vi "Host.vi"() -> ()   [LabVIEW 2018]
uses:
  <instrlib>/niDMM/nidmm.llb/niDMM Resolution in Digits.ctl
  <instrlib>/niDMM/nidmm.llb/niDMM Function.ctl
  <instrlib>/niDCPower/nidcpower.llb/niDCPower Measurement Type.ctl
  <instrlib>/niScope/Configure/Trigger/niScope Configure Trigger Edge.vi
  <instrlib>/niScope/Acquire/Fetch/niScope Multi Fetch Cluster.vi
  <instrlib>/niScope/Acquire/Fetch/niScope Fetch.vi
  <instrlib>/niDMM/nidmm.llb/niDMM Configure Measurement Digits.vi
panel:
  in  "Tab Control":enum32{"Панель управления", "Панель отладки"}(tab)
  out "Образец №":string="0"
  in  "SEL":path=path "D:/NI LabVIEW/21.057 MAX3738ETG+/SEL and SEU"
  out "VCC_char":dbl(graph)=6.67426339573744e-05
  in  "VCC, V":dbl=3.300000000000001 caption="voltage level" format="%_6p"
  out "VCC_cur, A":dbl=6.67426339573744e-05 caption="measurement" format="%_6g"
  in  "VCC_curlim, A":dbl=0.1 caption="current limit" format="%_6p"
  out "VCC_warning":bool
  in  "VCC_selcur, A":dbl=0.07 caption="current limit" format="%_6p"
  out "VCC_counter":u32
  out "SEL":bool
  out "SEU":bool
  in  "POWER":bool
  in  "Device Name":refnum<k15>="PXI1Slot6_3" caption="DMM (BIAS current)"
  in  "POWER (0 KEY(GND), 1 PRBS)":refnum<k15>="PXI1Slot3_3" caption="PRBS"
  in  "PRBS":bool
  in  "RELAY":bool
  in  "NI Scope (SHUTDOWN)":refnum<k15>="PXI1Slot5_2" caption="Scope"
  in  "POWER (0 VСС, 1 +5)":refnum<k15>="PXI1Slot2_2" caption="VСС_+5"
  out "DIOD, мA":dbl=0.00012235000212967861 caption="measurement" format="%_6g"
  out "SEU Waveform":T1(graph) caption="SHUTDOWN Waveform"
  in  "Trigger Level":dbl=2.9 format="%.2f"
  in  "Диапазон, A":dbl=0.1 caption="voltage level" format="%_6p"
  out "BC_MON_char":dbl(graph)=6.67426339573744e-05
  out "SEU_Counter":u32 caption="SEU counter"
  out "SEU_warning":bool caption="Find SEL"
  out "+5_char":dbl(graph)=4.2515020717360033e-07
  in  "+5, V":dbl=5.0 caption="voltage level" format="%_6p"
  out "+5_cur, A":dbl=4.2515020717360033e-07 caption="measurement" format="%_6g"
  in  "+5_curlim, A":dbl=0.1 caption="current limit" format="%_6p"
  out "PRBS_char":dbl(graph)=8.696388929340759e-07
  in  "PRBS, V":dbl=12.0 caption="voltage level" format="%_6p"
  out "PRBS_cur, A":dbl=8.696388929340759e-07 caption="measurement" format="%_6g"
  in  "PRBS_curlim, A":dbl=0.1 caption="current limit" format="%_6p"
  in  "SIM_SEL":bool
  in  "STOP":bool
  in  "Парирование SEU":bool=TRUE
  in  "Антизалип":bool=TRUE
  in  "POWER (0 DIOD, 1 TX_DISABLE)":refnum<k15>="PXI1Slot4_3" caption="PRBS"
  out "SHUTDOWN Waveform":T1(graph) caption="PC_MON Waveform"
  in  "DIOD_curlim, A":dbl=0.025 caption="current limit" format="%_6p"
  out "DIOD_cur, A":dbl=6.67426339573744e-05 caption="measurement" format="%_6g"
  in  "DIOD, V":dbl=3.300000000000001 caption="voltage level" format="%_6p"
  out "DIOD_char":dbl(graph)=6.67426339573744e-05
  in  "TX_DISABLE":bool
  in  "DIOD":bool
  in  "IN1(GND)":bool
  in  "IN1(GND)_curlim, A":dbl=0.01 caption="current limit" format="%_6p"
  out "IN1(GND)_cur, A":dbl=8.696388929340759e-07 caption="measurement" format="%_6g"
  in  "IN1(GND), V":dbl=3.3 caption="voltage level" format="%_6p"
  in  "TX_DISABLE_curlim, A":dbl=0.01 caption="current limit" format="%_6p"
  in  "TX_DISABLE, V":dbl=3.3 caption="voltage level" format="%_6p"
  out "TX_DISABLE_cur, A":dbl=8.696388929340759e-07 caption="measurement" format="%_6g"
  in  "SEU":path=path "D:/NI LabVIEW/21.057 MAX3738ETG+/SEL and SEU"
  out "Power OFF":bool
  in  "VCC ON":bool
  in  "Считать Ключ":bool
  in  "Считать SIM_SEL":bool
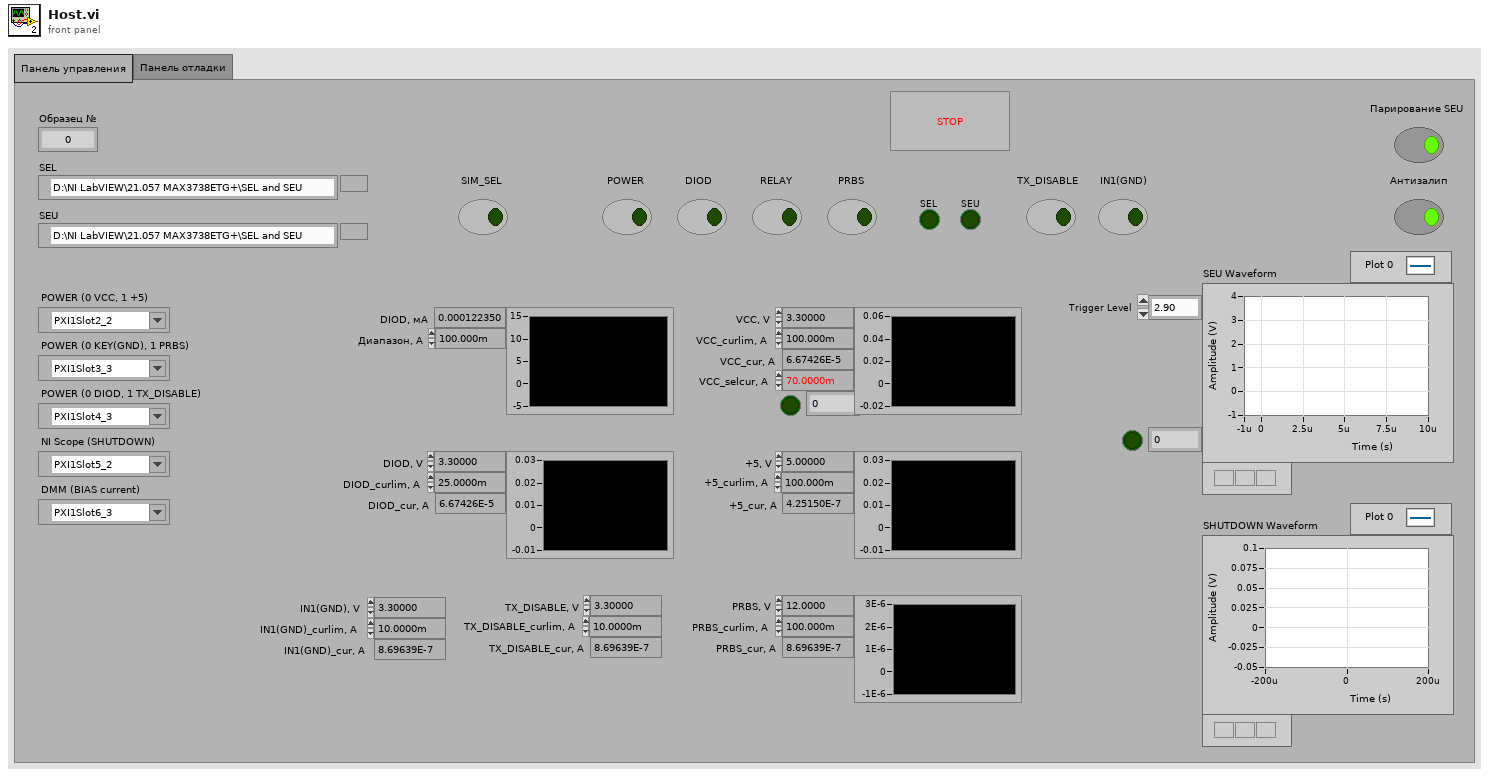
[diagram p1: front panel]
types:
  T1 = cluster{"relativeInitialX":dbl, "xIncrement":dbl, "wfm":dbl[]}[]
  T2 = enum16{"open", "replace", "create", "open or create", "replace or create", "replace or create with confirmation"}
  T3 = typedef "niDCPower Measurement Type.ctl" = i32
  T4 = typedef "niDMM Function.ctl" = enum16{"DC Volts", "AC Volts", "DC Current", "AC Current", "2-wire Resistance", "4-wire Resistance", "Diode", "Frequency", "Period", "AC Volts DC Coupled", "Capacitance", "Inductance", "Temperature"}
  T5 = typedef "niDMM Resolution in Digits.ctl" = dbl
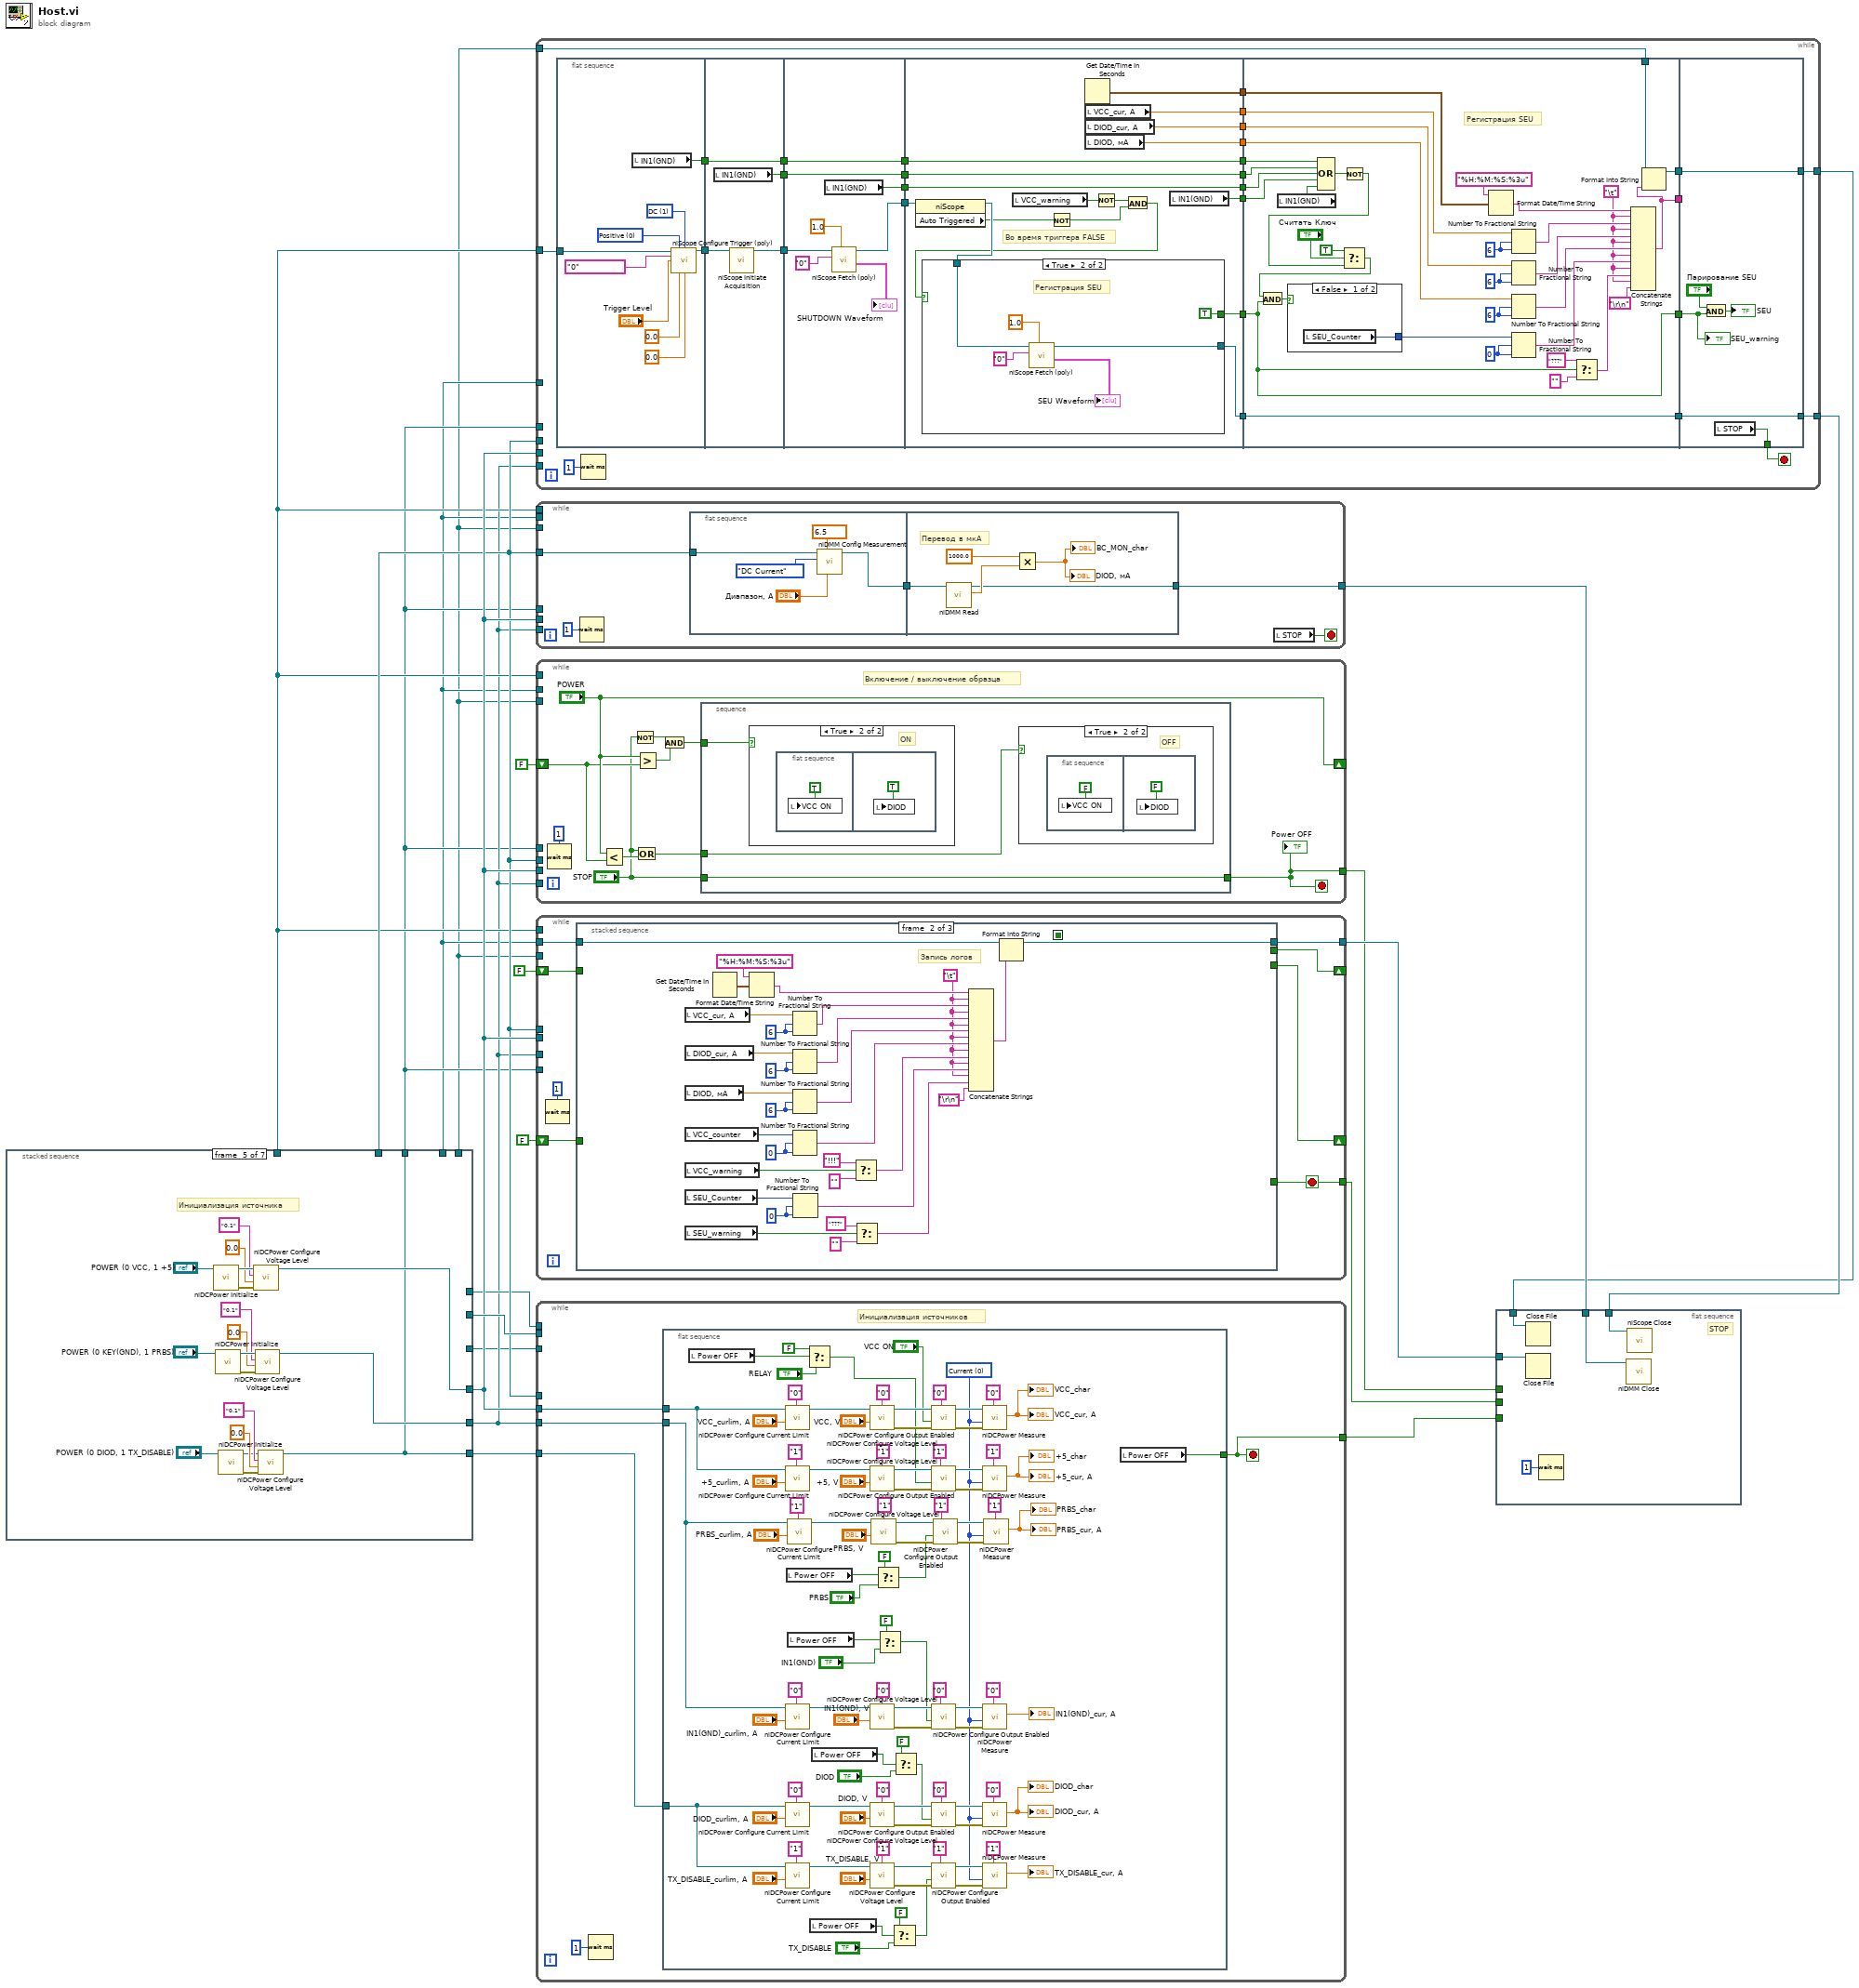
[diagram p0: block diagram]
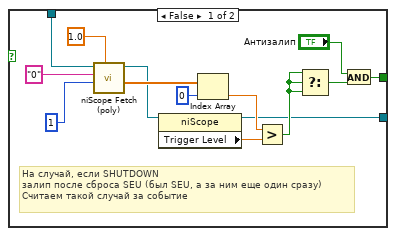
[diagram p2: hidden frame]
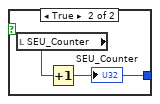
[diagram p3: hidden frame]
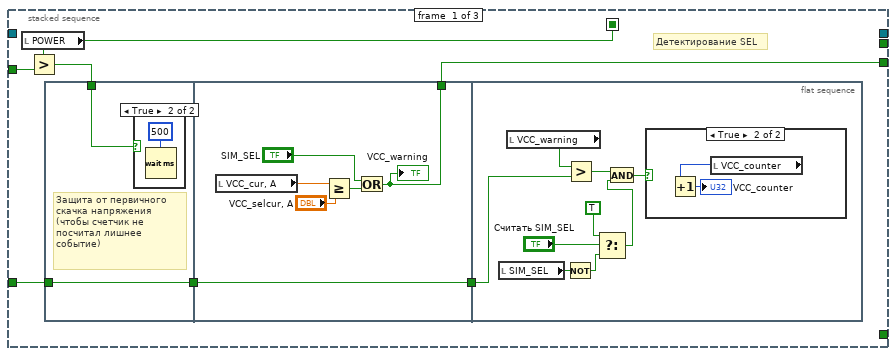
[diagram p4: hidden frame]
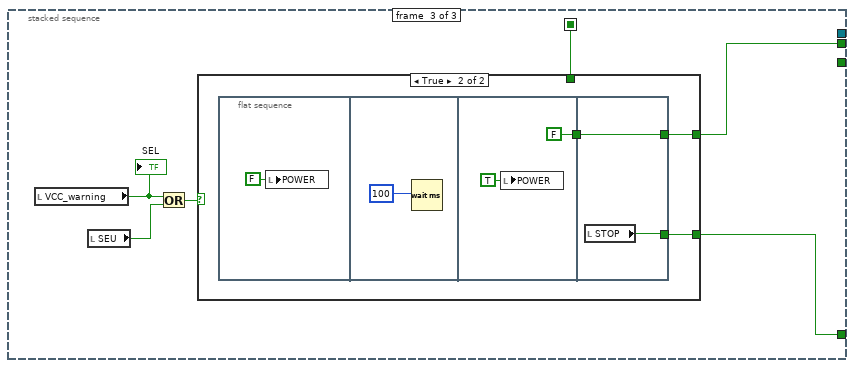
[diagram p7: hidden frame]
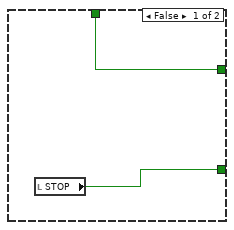
[diagram p8: hidden frame]
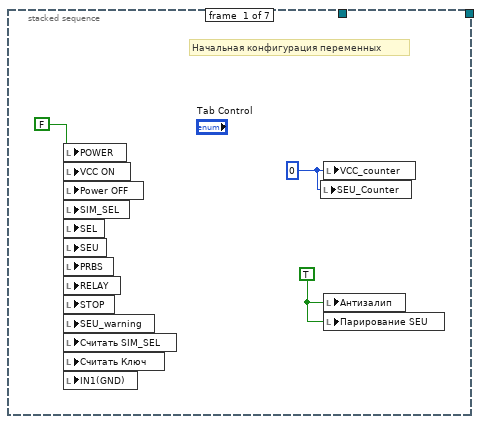
[diagram p11: hidden frame]
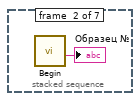
[diagram p12: hidden frame]
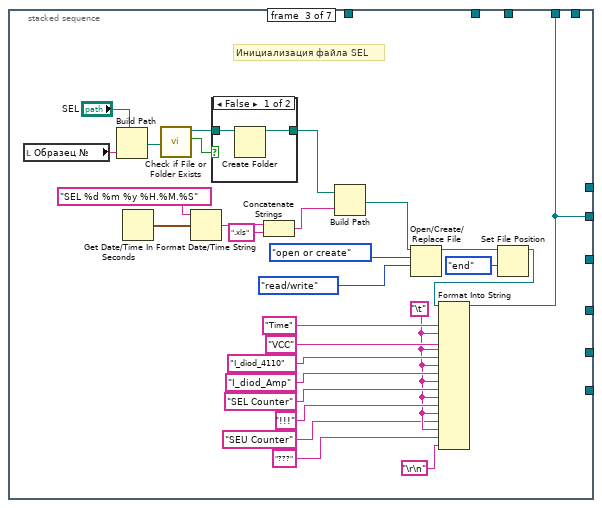
[diagram p13: hidden frame]
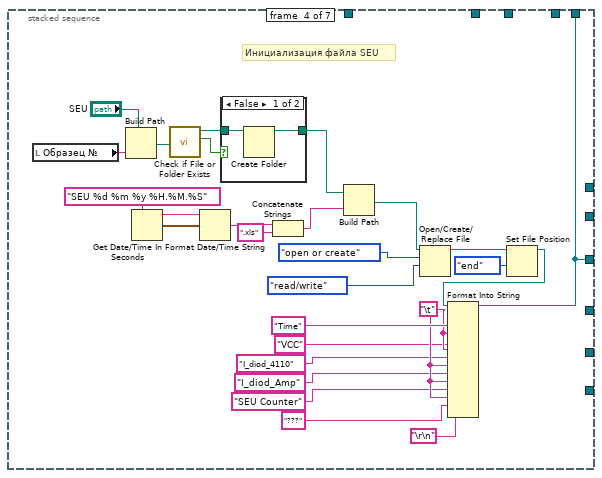
[diagram p15: hidden frame]
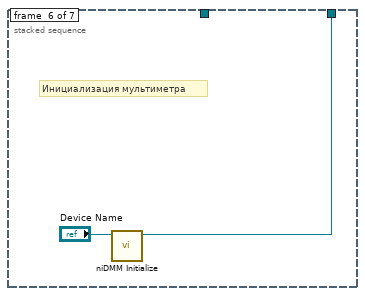
[diagram p17: hidden frame]
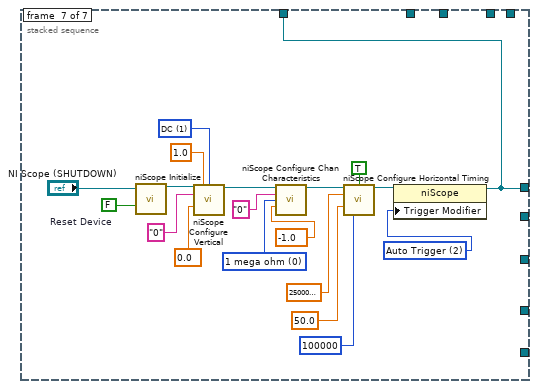
[diagram p18: hidden frame]
diagram:
  n1 = stacked-sequence {
    tunnel: [_ _ _ _ w99 _ _] -> w12
    tunnel: [_ _ w34 _ _ _ _] -> w4
    tunnel: [_ _ w34 _ _ _ _] -> w18
    tunnel: [_ _ _ _ _ w104 _] -> w11
    tunnel: [_ _ _ _ w92 _ _] -> w7
    tunnel: [_ _ _ _ _ _ w106] -> w10
    tunnel: [_ _ _ _ _ _ w106] -> w9
    tunnel: [_ _ _ _ w86 _ _] -> w6
    tunnel: [_ _ _ _ w86 _ _] -> w5
    tunnel: [_ _ _ w57 _ _ _] -> w3
    tunnel: [_ _ _ w57 _ _ _] -> w2
    frame #0 {
      w23 = TRUE ("Питание")
      w24 = u32 0 ("VCC_counter")
      w22 = FALSE ("Питание")
      # "Начальная конфигурация переменных"
      n2 = local write "POWER"(w22) -> ()
      n3 = local write "VCC ON"(w22) -> ()
      n4 = local write "Power OFF"(w22) -> ()
      n5 = local write "SIM_SEL"(w22) -> ()
      n6 = local write "SEL"(w22) -> ()
      n7 = local write "SEU"(w22) -> ()
      n8 = local write "PRBS"(w22) -> ()
      n9 = local write "RELAY"(w22) -> ()
      n10 = local write "STOP"(w22) -> ()
      n11 = local write "SEU_warning"(w22) -> ()
      n12 = local write "Считать SIM_SEL"(w22) -> ()
      n13 = local write "Считать Ключ"(w22) -> ()
      n14 = local write "IN1(GND)"(w22) -> ()
      n15 = local write "SEU_Counter"(w24) -> ()
      n16 = local write "VCC_counter"(w24) -> ()
      n17 = local write "Антизалип"(w23) -> ()
      n18 = local write "Парирование SEU"(w23) -> ()
    }
    frame #1 {
      n19 = call "Begin.vi"() -> ("Образец № 2"=→"Образец №":string)  [unwired: 9 in]
    }
    frame #2 {
      w29 = "\t"
      # "Инициализация файла SEL"
      n20 = local read "Образец №"() -> (w36:string)
      n21 = Build Path(base path="SEL", name or relative path=w36) -> (appended path=w53:path)
      n22 = Get Date/Time In Seconds() -> (seconds since 1Jan1904=w49:timestamp)
      n23 = call <vilib>:"Check if File or Folder Exists.vi"("path"=w53) -> ("file or folder exists?"=w52:bool, "dup path"=w51:path)  [unwired: 8 in, 1 out]
      n24 = Format Date/Time String(time format string (%c)="SEL %d %m %y %H.%M.%S", seconds (now)=w49) -> (date/time string=w48:string)  [unwired: 1 in]
      n25 = case shown="False" w52 {
        tunnel: w51 -> [w55 w56]
        tunnel: [w54 w56] -> w50
        frame False {
          n26 = Create Folder(path (use dialog)=w55) -> (created path=w54:path)  [unwired: 2 in, 2 out]
        }
        frame True {
        }
      }
      n27 = Concatenate Strings(w48, ".xls" ("string")) -> (w45:string)
      n28 = Build Path(base path=w50, name or relative path=w45) -> (appended path=w42:path)
      n29 = Open/Create/Replace File(file path (use dialog)=w42, operation (0:open)=T2."open or create", access (0:read/write)=enum16{"read/write", "read-only", "write-only"}."read/write") -> (refnum out=w39:refnum<file>)  [unwired: 3 in, 2 out]
      n30 = Set File Position(refnum=w39, from (0:start)=enum16{"start", "end", "current"}."end") -> (refnum out=w35:refnum<file>)  [unwired: 2 in, 1 out]
      n31 = Format Into String(initial string=w35, "Time" ("string"), w29, "VCC" ("string"), w29, "I_diod_4110" ("string"), w29, "I_diod_Amp" ("input 7"), w29, "SEL Counter" ("string"), w29, "!!!" ("string"), w29, "SEU Counter" ("string"), w29, "???" ("string"), "\r\n") -> (resulting string=w34:refnum<file>)  [unwired: 2 in, 1 out]
    }
    frame #3 {
      w69 = "\t"
      # "Инициализация файла SEU"
      n32 = local read "Образец №"() -> (w72:string)
      n33 = Build Path(base path="SEU", name or relative path=w72) -> (appended path=w82:path)
      n34 = Get Date/Time In Seconds() -> (seconds since 1Jan1904=w78:timestamp)
      n35 = call <vilib>:"Check if File or Folder Exists.vi"("path"=w82) -> ("file or folder exists?"=w81:bool, "dup path"=w80:path)  [unwired: 8 in, 1 out]
      n36 = Format Date/Time String(time format string (%c)="SEU %d %m %y %H.%M.%S", seconds (now)=w78) -> (date/time string=w77:string)  [unwired: 1 in]
      n37 = case shown="False" w81 {
        tunnel: w80 -> [w84 w85]
        tunnel: [w83 w85] -> w79
        frame False {
          n38 = Create Folder(path (use dialog)=w84) -> (created path=w83:path)  [unwired: 2 in, 2 out]
        }
        frame True {
        }
      }
      n39 = Concatenate Strings(w77, ".xls" ("string")) -> (w76:string)
      n40 = Build Path(base path=w79, name or relative path=w76) -> (appended path=w75:path)
      n41 = Open/Create/Replace File(file path (use dialog)=w75, operation (0:open)=T2."open or create", access (0:read/write)=enum16{"read/write", "read-only", "write-only"}."read/write") -> (refnum out=w74:refnum<file>)  [unwired: 3 in, 2 out]
      n42 = Set File Position(refnum=w74, from (0:start)=enum16{"start", "end", "current"}."end") -> (refnum out=w58:refnum<file>)  [unwired: 2 in, 1 out]
      n43 = Format Into String(initial string=w58, "Time" ("string"), w69, "VCC" ("string"), w69, "I_diod_4110" ("string"), w69, "I_diod_Amp" ("input 7"), w69, "SEU Counter" ("string"), w69, "???" ("string"), "\r\n") -> (resulting string=w57:refnum<file>)  [unwired: 2 in, 1 out]
    }
    frame #4 {
      # "Инициализация источника"
      n44 = call <instrlib>:"niDCPower Initialize.vi"("resource name"="POWER (0 VСС, 1 +5)") -> ("error out"=w102:errorcluster, "instrument handle out"=w103:refnum<k15>)  [unwired: 3 in, 6 out]
      n45 = call <instrlib>:"niDCPower Initialize.vi"("resource name"="POWER (0 KEY(GND), 1 PRBS)") -> ("error out"=w96:errorcluster, "instrument handle out"=w97:refnum<k15>)  [unwired: 3 in, 6 out]
      n46 = call <instrlib>:"niDCPower Initialize.vi"("resource name"="POWER (0 DIOD, 1 TX_DISABLE)") -> ("error out"=w88:errorcluster, "instrument handle out"=w87:refnum<k15>)  [unwired: 3 in, 6 out]
      n47 = call <instrlib>:"niDCPower Configure Voltage Level.vi"("error in (no error)"=w102, "voltage level"=0.0, "channel name"="0,1", "instrument handle"=w103) -> ("instrument handle out"=w99:refnum<k15>)  [unwired: 6 in, 1 out]
      n48 = call <instrlib>:"niDCPower Configure Voltage Level.vi"("error in (no error)"=w96, "voltage level"=0.0, "channel name"="0,1", "instrument handle"=w97) -> ("instrument handle out"=w92:refnum<k15>)  [unwired: 6 in, 1 out]
      n49 = call <instrlib>:"niDCPower Configure Voltage Level.vi"("error in (no error)"=w88, "voltage level"=0.0, "channel name"="0,1", "instrument handle"=w87) -> ("instrument handle out"=w86:refnum<k15>)  [unwired: 6 in, 1 out]
    }
    frame #5 {
      # "Инициализация мультиметра"
      n50 = call <instrlib>:"niDMM Initialize.vi"("Instrument Descriptor"="Device Name") -> ("instrument handle out"=w104:refnum<k15>)  [unwired: 9 in, 1 out]
    }
    frame #6 {
      w109 = 2 items=["None"=1, "Auto Trigger"=2] ("Triggering:Trigger Modifier")
      w116 = u32 0 items=["1 mega ohm"=0, "50 ohms"=2] ("Input Impedance")
      w121 = 1 items=["AC", "DC", "Ground"] ("Vertical Coupling")
      w123 = FALSE  # Reset Device
      n51 = call <instrlib>:"niScope Initialize.vi"("resource name"="NI Scope (SHUTDOWN)", "reset device"=w123) -> ("instrument handle"=w118:refnum<k15>)  [unwired: 12 in, 1 out]
      n52 = call <instrlib>:"niScope Configure Vertical.vi"("instrument handle"=w118, "probe attenuation"=1.0 ("Probe Attenuation"), "vertical coupling"=w121, "channels"="0" ("Channel Name"), "vertical offset"=0.0 ("Vertical Offset")) -> ("instrument handle out"=w114:refnum<k15>)  [unwired: 9 in, 1 out]
      n53 = call <instrlib>:"niScope Configure Chan Characteristics.vi"("instrument handle"=w114, "channels"="0" ("Channel Name"), "input impedance"=w116, "maximum input frequency"=-1.0 ("Maximum Input Frequency")) -> ("instrument handle out"=w108:refnum<k15>)  [unwired: 10 in, 1 out]
      n54 = call <instrlib>:"niScope Configure Horizontal Timing.vi"("instrument handle"=w108, "enforce realtime"=TRUE ("Enforce Realtime"), "min sample rate"=250000000.0 ("Min Sample Rate"), "reference position"=50.0 ("Reference\nPosition"), "min record length"=100000 ("Min Record Length")) -> ("instrument handle out"=w107:refnum<k15>)  [unwired: 9 in, 1 out]
      n55 = property on="Property Node" class="niScope"(reference=w107, "Trigger Modifier"=w109) -> (reference out=w106:refnum<k15>)  [unwired: 1 in, 1 out]
    }
  }
  n56 = while {
    tunnel: w12 -> [w129]
    tunnel: [w128] -> w16
    tunnel: w18 -> [_]
    tunnel: w7 -> [w127]
    tunnel: w11 -> [_]
    tunnel: w9 -> [_]
    tunnel: w6 -> [w125]
    tunnel: w3 -> [_]
    stop <- w128 stop-if-true
    # "Инициализация источников"
    n57 = Wait (ms)(milliseconds to wait=u32 1) -> ()  [unwired: 1 out]
    n58 = flat-sequence {
      tunnel: w129 -> [w227]
      tunnel: [w202] -> w128
      tunnel: w127 -> [w145]
      tunnel: w125 -> [w144]
      frame #0 {
        w143 = T3 0 items=["Current", "Voltage"] ("measurement type")
        n59 = local read "Power OFF"() -> (w187:bool)
        n60 = call <instrlib>:"niDCPower Configure Current Limit.vi"("current limit"="VCC_curlim, A", "channel name"="0", "instrument handle"=w227) -> ("instrument handle out"=w216:refnum<k15>)  [unwired: 7 in, 1 out]
        n61 = call <instrlib>:"niDCPower Configure Current Limit.vi"("current limit"="+5_curlim, A", "channel name"="1", "instrument handle"=w227) -> ("instrument handle out"=w213:refnum<k15>)  [unwired: 7 in, 1 out]
        n62 = call <instrlib>:"niDCPower Configure Current Limit.vi"("current limit"="IN1(GND)_curlim, A", "channel name"="0", "instrument handle"=w145) -> ("instrument handle out"=w174:refnum<k15>)  [unwired: 7 in, 1 out]
        n63 = call <instrlib>:"niDCPower Configure Current Limit.vi"("current limit"="DIOD_curlim, A", "channel name"="0", "instrument handle"=w144) -> ("instrument handle out"=w156:refnum<k15>)  [unwired: 7 in, 1 out]
        n64 = call <instrlib>:"niDCPower Configure Current Limit.vi"("current limit"="TX_DISABLE_curlim, A", "channel name"="1", "instrument handle"=w144) -> ("instrument handle out"=w158:refnum<k15>)  [unwired: 7 in, 1 out]
        n65 = local read "Power OFF"() -> (w188:bool)
        n66 = call <instrlib>:"niDCPower Configure Current Limit.vi"("current limit"="PRBS_curlim, A", "channel name"="1", "instrument handle"=w145) -> ("instrument handle out"=w196:refnum<k15>)  [unwired: 7 in, 1 out]
        n67 = local read "Power OFF"() -> (w138:bool)
        n68 = Select(t=FALSE, s=w187, f="RELAY") -> (s? t:f=w184:bool)
        n69 = local read "Power OFF"() -> (w133:bool)
        n70 = local read "Power OFF"() -> (w141:bool)
        n71 = call <instrlib>:"niDCPower Configure Voltage Level.vi"("voltage level"="VCC, V", "channel name"="0", "instrument handle"=w216) -> ("error out"=w221:errorcluster, "instrument handle out"=w222:refnum<k15>)  [unwired: 7 in]
        n72 = call <instrlib>:"niDCPower Configure Voltage Level.vi"("voltage level"="+5, V", "channel name"="1", "instrument handle"=w213) -> ("error out"=w219:errorcluster, "instrument handle out"=w220:refnum<k15>)  [unwired: 7 in]
        n73 = call <instrlib>:"niDCPower Configure Voltage Level.vi"("voltage level"="IN1(GND), V", "channel name"="0", "instrument handle"=w174) -> ("error out"=w172:errorcluster, "instrument handle out"=w171:refnum<k15>)  [unwired: 7 in]
        n74 = call <instrlib>:"niDCPower Configure Voltage Level.vi"("voltage level"="DIOD, V", "channel name"="0", "instrument handle"=w156) -> ("error out"=w151:errorcluster, "instrument handle out"=w150:refnum<k15>)  [unwired: 7 in]
        n75 = call <instrlib>:"niDCPower Configure Voltage Level.vi"("voltage level"="TX_DISABLE, V", "channel name"="1", "instrument handle"=w158) -> ("error out"=w153:errorcluster, "instrument handle out"=w152:refnum<k15>)  [unwired: 7 in]
        n76 = call <instrlib>:"niDCPower Configure Voltage Level.vi"("voltage level"="PRBS, V", "channel name"="1", "instrument handle"=w196) -> ("error out"=w198:errorcluster, "instrument handle out"=w199:refnum<k15>)  [unwired: 7 in]
        n77 = Select(t=FALSE, s=w188, f="PRBS") -> (s? t:f=w181:bool)
        n78 = Select(t=FALSE, s=w138, f="IN1(GND)") -> (s? t:f=w136:bool)
        n79 = Select(t=FALSE, s=w133, f="TX_DISABLE") -> (s? t:f=w131:bool)
        n80 = Select(t=FALSE, s=w141, f="DIOD") -> (s? t:f=w140:bool)
        n81 = call <instrlib>:"niDCPower Configure Output Enabled.vi"("error in (no error)"=w221, "output enabled"="VCC ON", "channel name"="0", "instrument handle"=w222) -> ("error out"=w224:errorcluster, "instrument handle out"=w223:refnum<k15>)  [unwired: 6 in]
        n82 = call <instrlib>:"niDCPower Configure Output Enabled.vi"("error in (no error)"=w219, "output enabled"=w184, "channel name"="1", "instrument handle"=w220) -> ("error out"=w226:errorcluster, "instrument handle out"=w225:refnum<k15>)  [unwired: 6 in]
        n83 = call <instrlib>:"niDCPower Configure Output Enabled.vi"("error in (no error)"=w172, "output enabled"=w136, "channel name"="0", "instrument handle"=w171) -> ("error out"=w169:errorcluster, "instrument handle out"=w170:refnum<k15>)  [unwired: 6 in]
        n84 = call <instrlib>:"niDCPower Configure Output Enabled.vi"("error in (no error)"=w151, "output enabled"=w140, "channel name"="0", "instrument handle"=w150) -> ("error out"=w148:errorcluster, "instrument handle out"=w149:refnum<k15>)  [unwired: 6 in]
        n85 = call <instrlib>:"niDCPower Configure Output Enabled.vi"("error in (no error)"=w153, "output enabled"=w131, "channel name"="1", "instrument handle"=w152) -> ("error out"=w146:errorcluster, "instrument handle out"=w147:refnum<k15>)  [unwired: 6 in]
        n86 = call <instrlib>:"niDCPower Configure Output Enabled.vi"("error in (no error)"=w198, "output enabled"=w181, "channel name"="1", "instrument handle"=w199) -> ("error out"=w201:errorcluster, "instrument handle out"=w200:refnum<k15>)  [unwired: 6 in]
        n87 = call <instrlib>:"niDCPower Measure.vi"("error in (no error)"=w224, "measurement type"=w143, "channel name"="0", "instrument handle"=w223) -> ("measurement"=→"VCC_cur, A" →"VCC_char":dbl)  [unwired: 5 in, 2 out]
        n88 = call <instrlib>:"niDCPower Measure.vi"("error in (no error)"=w226, "measurement type"=w143, "channel name"="1", "instrument handle"=w225) -> ("measurement"=→"+5_cur, A" →"+5_char":dbl)  [unwired: 5 in, 2 out]
        n89 = call <instrlib>:"niDCPower Measure.vi"("error in (no error)"=w169, "measurement type"=w143, "channel name"="0", "instrument handle"=w170) -> ("measurement"=→"IN1(GND)_cur, A":dbl)  [unwired: 5 in, 2 out]
        n90 = call <instrlib>:"niDCPower Measure.vi"("error in (no error)"=w148, "measurement type"=w143, "channel name"="0", "instrument handle"=w149) -> ("measurement"=→"DIOD_cur, A" →"DIOD_char":dbl)  [unwired: 5 in, 2 out]
        n91 = call <instrlib>:"niDCPower Measure.vi"("error in (no error)"=w146, "measurement type"=w143, "channel name"="1", "instrument handle"=w147) -> ("measurement"=→"TX_DISABLE_cur, A":dbl)  [unwired: 5 in, 2 out]
        n92 = call <instrlib>:"niDCPower Measure.vi"("error in (no error)"=w201, "measurement type"=w143, "channel name"="1", "instrument handle"=w200) -> ("measurement"=→"PRBS_cur, A" →"PRBS_char":dbl)  [unwired: 5 in, 2 out]
        n93 = local read "Power OFF"() -> (w202:bool)
      }
    }
  }
  n94 = while {
    tunnel: w10 -> [w251]
    tunnel: w12 -> [_]
    tunnel: w7 -> [_]
    tunnel: w11 -> [_]
    tunnel: [w256] -> w8
    tunnel: w5 -> [_]
    tunnel: w4 -> [_]
    tunnel: w2 -> [w235]
    tunnel: [w233] -> w1
    stop <- w252 stop-if-true
    n95 = flat-sequence {
      tunnel: [w259] -> w255
      tunnel: w251 -> [w258]
      tunnel: [w257] -> w244
      tunnel: [w269] -> w254
      tunnel: w255 -> [w268]
      tunnel: [w267] -> w248
      tunnel: [w266] -> w245
      tunnel: w244 -> [w266]
      tunnel: w254 -> [w274]
      tunnel: [w273] -> w253
      tunnel: [w272] -> w249
      tunnel: w248 -> [w271]
      tunnel: [w271] -> w247
      tunnel: [w270] -> w246
      tunnel: w245 -> [w270]
      tunnel: [w292] -> w243
      tunnel: w253 -> [w294]
      tunnel: [w291] -> w241
      tunnel: [w285] -> w240
      tunnel: [w284] -> w239
      tunnel: w249 -> [w284]
      tunnel: [w283] -> w238
      tunnel: w247 -> [w283]
      tunnel: [w282] -> w237
      tunnel: w246 -> [w282]
      tunnel: [w281] -> w231
      tunnel: [w280] -> w230
      tunnel: [w279] -> w229
      tunnel: [w278] -> w228
      tunnel: w243 -> [w350]
      tunnel: [w350] -> w242
      tunnel: w241 -> [w321]
      tunnel: w240 -> [w325]
      tunnel: w239 -> [w326]
      tunnel: w238 -> [w327]
      tunnel: w237 -> [w328]
      tunnel: [w321] -> w236
      tunnel: w235 -> [w336]
      tunnel: [w335] -> w234
      tunnel: [w319] -> w232
      tunnel: w231 -> [w318]
      tunnel: w230 -> [w317]
      tunnel: w229 -> [w316]
      tunnel: w228 -> [w315]
      tunnel: [w356] -> w256
      tunnel: w242 -> [w356]
      tunnel: [w358] -> w252
      tunnel: w236 -> [w355]
      tunnel: w234 -> [w354]
      tunnel: [w354] -> w233
      tunnel: w232 -> [_]
      frame #0 {
        w264 = 0 items=["Positive", "Negative"] ("Trigger Slope")
        w263 = u16 1 items=["AC"=0, "DC"=1, "HF Reject"=3, "LF Reject"=4, "AC Plus HF Reject"=1001] ("Coupling")
        n96 = local read "IN1(GND)"() -> (w257:bool)
        n97 = call-poly <instrlib>:"niScope Configure Trigger (poly).vi"("instrument handle"=w258, "trigger slope"=w264, "trigger coupling"=w263, "trigger source"="0" ("Trigger Source"), "trigger level"="Trigger Level", "trigger holdoff"=0.0, "trigger delay"=0.0 ("Trigger Delay")) -> ("instrument handle out"=w259:refnum<k15>)  [unwired: 7 in, 1 out]
      }
      frame #1 {
        n98 = local read "IN1(GND)"() -> (w267:bool)
        n99 = call <instrlib>:"niScope Initiate Acquisition.vi"("instrument handle"=w268) -> ("instrument handle out"=w269:refnum<k15>)  [unwired: 13 in, 1 out]
      }
      frame #2 {
        n100 = local read "IN1(GND)"() -> (w272:bool)
        n101 = call-poly <instrlib>:"niScope Fetch (poly).vi"("timeout"=1.0, "channels"="0", "instrument handle"=w274) -> ("waveform"=→"SHUTDOWN Waveform":T1, "instrument handle out"=w273:refnum<k15>)  [unwired: 5 in, 2 out]
      }
      frame #3 {
        # "Во время триггера FALSE"
        n102 = property class="niScope"(reference=w294) -> (reference out=w293:refnum<k15>, "Auto Triggered"=w290:bool)  [unwired: 1 in, 1 out]
        n103 = local read "VCC_warning"() -> (w286:bool)
        n104 = Not(x=w290) -> (.not. x?=w289:bool)
        n105 = Get Date/Time In Seconds() -> (seconds since 1Jan1904=w281:timestamp)
        n106 = local read "VCC_cur, A"() -> (w278:dbl)
        n107 = local read "DIOD_cur, A"() -> (w279:dbl)
        n108 = local read "DIOD, мA"() -> (w280:dbl)
        n109 = Not(x=w286) -> (.not. x?=w287:bool)
        n110 = And(x=w287, y=w289) -> (x .and. y?=w288:bool)
        n111 = case shown="True" w288 {
          tunnel: w293 -> [w306 w311]
          tunnel: [w299 w310] -> w292
          tunnel: [w298 TRUE] -> w291
          frame False {
            # "На случай, если SHUTDOWN\nзалип после сброса SEU (был SEU, а за ним еще один сразу)\nСчитаем такой случай за событие"
            n112 = call-poly <instrlib>:"niScope Fetch (poly).vi"("timeout"=1.0, "numSamples"=1, "channels"="0", "instrument handle"=w306) -> ("wfm"=w305:dbl[], "instrument handle out"=w300:refnum<k15>)  [unwired: 4 in, 2 out]
            n113 = property class="niScope"(reference=w300) -> (reference out=w299:refnum<k15>, "Trigger Level"=w302:dbl)  [unwired: 1 in, 1 out]
            n114 = Index Array(array=w305, index=0) -> (element=w303:dbl)
            n115 = Greater?(x=w303, y=w302) -> (0:w301:bool)
            n116 = Select(t=w301, s=w301, f=w301) -> (s? t:f=w297:bool)
            n117 = And(x="Антизалип", y=w297) -> (x .and. y?=w298:bool)
          }
          frame True {
            # "Регистрация SEU"
            n118 = call-poly <instrlib>:"niScope Fetch (poly).vi"("timeout"=1.0, "channels"="0", "instrument handle"=w311) -> ("waveform"=→"SEU Waveform":T1, "instrument handle out"=w310:refnum<k15>)  [unwired: 5 in, 2 out]
          }
        }
        n119 = local read "IN1(GND)"() -> (w285:bool)
      }
      frame #4 {
        w338 = 6
        w343 = 6
        w342 = 6
        w339 = 0
        w334 = "\t"
        # "Регистрация SEU"
        n120 = local read "IN1(GND)"() -> (w332:bool)
        n121 = Compound Arithmetic op=OR(w328, w327, w326, w325, w332) -> (w331:bool)
        n122 = Not(x=w331) -> (.not. x?=w323:bool)
        n123 = Select(t=TRUE, s="Считать Ключ", f=w323) -> (s? t:f=w320:bool)
        n124 = And(x=w320, y=w321) -> (x .and. y?=w322:bool)
        n125 = case shown="False" w322 {
          tunnel: [w351 w352] -> w324
          frame False {
            n126 = local read "SEU_Counter"() -> (w351:u32)
          }
          frame True {
            n127 = local read "SEU_Counter"() -> (w353:u32)
            n128 = Increment(x=w353) -> (x+1=w352:u32)
            "SEU_Counter" <- w352
          }
        }
        n129 = Format Date/Time String(time format string (%c)="%H:%M:%S:%3u", seconds (now)=w318) -> (date/time string=w345:string)  [unwired: 1 in]
        n130 = Number To Fractional String(number=w315, width (-)=w338, precision (6)=w338) -> (F-format string=w344:string)  [unwired: 1 in]
        n131 = Number To Fractional String(number=w316, width (-)=w342, precision (6)=w342) -> (F-format string=w346:string)  [unwired: 1 in]
        n132 = Number To Fractional String(number=w317, width (-)=w343, precision (6)=w343) -> (F-format string=w347:string)  [unwired: 1 in]
        n133 = Number To Fractional String(number=w324, width (-)=w339, precision (6)=w339) -> (F-format string=w348:string)  [unwired: 1 in]
        n134 = Select(t="???", s=w321, f="") -> (s? t:f=w349:string)
        n135 = Concatenate Strings(w345, w334, w344, w334, w346, w334, w347, w334, w348, w334, w349, w334, "\r\n") -> (w319:string)
        n136 = Format Into String(initial string=w336, w319) -> (resulting string=w335:refnum<file>)  [unwired: 2 in, 1 out]
      }
      frame #5 {
        n137 = And(x="Парирование SEU", y=w355) -> (x .and. y?=→"SEU":bool)
        n138 = local read "STOP"() -> (w358:bool)
        "SEU_warning" <- w355
      }
    }
    n139 = Wait (ms)(milliseconds to wait=u32 1) -> ()  [unwired: 1 out]
  }
  n140 = while {
    tunnel: w11 -> [w360]
    tunnel: [w364] -> w13
    tunnel: w4 -> [_]
    tunnel: w12 -> [_]
    tunnel: w7 -> [_]
    tunnel: w10 -> [_]
    tunnel: w5 -> [_]
    tunnel: w2 -> [_]
    stop <- w363 stop-if-true
    n141 = Wait (ms)(milliseconds to wait=u32 1) -> ()  [unwired: 1 out]
    n142 = flat-sequence {
      tunnel: [w367] -> w361
      tunnel: w360 -> [w366]
      tunnel: [w370] -> w364
      tunnel: w361 -> [w374]
      frame #0 {
        w369 = T5 6.5 items=["3 1/2"=3.5, "4 1/2"=4.5, "5 1/2"=5.5, "6 1/2"=6.5, "7 1/2"=7.5] ("Resolution in Digits")
        n143 = call-poly <instrlib>:"niDMM Config Measurement.vi"("Range"="Диапазон, A", "Resolution in Digits"=w369, "Function"=niDMM_Function."DC Current" ("Measurement Type"), "instrument handle"=w366) -> ("instrument handle out"=w367:refnum<k15>)  [unwired: 6 in, 1 out]
      }
      frame #1 {
        # "Перевод в мкА"
        n144 = call <instrlib>:"niDMM Read.vi"("instrument handle"=w374) -> ("Measurement"=w372:dbl, "instrument handle out"=w370:refnum<k15>)  [unwired: 8 in, 1 out]
        n145 = Multiply(x=1000.0 ("y"), y=w372) -> (x*y=→"DIOD, мA" →"BC_MON_char":dbl)
      }
    }
    n146 = local read "STOP"() -> (w363:bool)
  }
  n147 = while {
    shift-right: ["POWER"] -> _
    shift-left: FALSE ("Питание") -> [w383]
    tunnel: [w375] -> w14
    tunnel: w4 -> [_]
    tunnel: w12 -> [_]
    tunnel: w7 -> [_]
    tunnel: w11 -> [_]
    tunnel: w10 -> [_]
    tunnel: w5 -> [_]
    tunnel: w2 -> [_]
    stop <- w375 stop-if-true
    # "Включение / выключение образца"
    n148 = Wait (ms)(milliseconds to wait=u32 1) -> ()  [unwired: 1 out]
    n149 = Less?(x="POWER", y=w383) -> (x < y?=w378:bool)
    n150 = Not(x="STOP") -> (.not. x?=w380:bool)
    n151 = Or(x="STOP", y=w378) -> (x .or. y?=w377:bool)
    n152 = Greater?(x="POWER", y=w383) -> (0:w379:bool)
    n153 = And(x=w380, y=w379) -> (x .and. y?=w381:bool)
    n154 = stacked-sequence {
      tunnel: w381 -> [w387]
      tunnel: w377 -> [w385]
      tunnel: [w386] -> w375
      tunnel: "STOP" -> [w386]
      frame #0 {
        n155 = case shown="True" w387 {
          frame False {
          }
          frame True {
            # "ON"
            n156 = flat-sequence {
              frame #0 {
                n157 = local write "VCC ON"(TRUE ("VDD18_ON")) -> ()
              }
              frame #1 {
                n158 = local write "DIOD"(TRUE ("VDD18_ON")) -> ()
              }
            }
          }
        }
        n159 = case shown="True" w385 {
          frame False {
          }
          frame True {
            # "OFF"
            n160 = flat-sequence {
              frame #0 {
                n161 = local write "VCC ON"(FALSE ("VDD18_ON")) -> ()
              }
              frame #1 {
                n162 = local write "DIOD"(FALSE ("VDD18_ON")) -> ()
              }
            }
          }
        }
      }
    }
    "Power OFF" <- w375
  }
  n163 = while {
    shift-right: [w392] -> _
    shift-left: FALSE ("Питание") -> [w399]
    tunnel: w4 -> [w397]
    tunnel: [w396] -> w15
    tunnel: [w395] -> w17
    shift-right: [w393] -> _
    shift-left: FALSE ("Питание") -> [w394]
    tunnel: w12 -> [_]
    tunnel: w7 -> [_]
    tunnel: w11 -> [_]
    tunnel: w10 -> [_]
    tunnel: w5 -> [_]
    tunnel: w2 -> [_]
    stop <- w396 stop-if-true
    n164 = Wait (ms)(milliseconds to wait=u32 1) -> ()  [unwired: 1 out]
    n165 = stacked-sequence {
      seq-local: [w400 _ _] -> [_ _ w461]
      tunnel: w399 -> [w406 _ _]
      tunnel: [_ _ w463] -> w396
      tunnel: w397 -> [_ w446 _]
      tunnel: [_ w445 _] -> w395
      tunnel: w394 -> [w403 _ _]
      tunnel: [w401 _ _] -> w393
      tunnel: [_ _ w462] -> w392
      frame #0 {
        # "Детектирование SEL"
        n166 = local read "POWER"() -> (w400:bool)
        n167 = Greater?(x=w400, y=w406) -> (0:w405:bool)
        n168 = flat-sequence {
          tunnel: w405 -> [w407]
          tunnel: [w408] -> w404
          tunnel: w403 -> [w408]
          tunnel: [w412] -> w401
          tunnel: w404 -> [w411]
          tunnel: [w411] -> w402
          tunnel: w402 -> [w420]
          frame #0 {
            # "Защита от первичного скачка напряжения\n(чтобы счетчик не посчитал лишнее событие)"
            n169 = case shown="True" w407 {
              frame False {
              }
              frame True {
                n170 = Wait (ms)(milliseconds to wait=u32 500) -> ()  [unwired: 1 out]
              }
            }
          }
          frame #1 {
            n171 = local read "VCC_cur, A"() -> (w415:dbl)
            n172 = Greater Or Equal?(x=w415, y="VCC_selcur, A") -> (x >= y?=w413:bool)
            n173 = Or(x="SIM_SEL", y=w413) -> (x .or. y?=w412:bool)
            "VCC_warning" <- w412
          }
          frame #2 {
            n174 = local read "SIM_SEL"() -> (w422:bool)
            n175 = local read "VCC_warning"() -> (w421:bool)
            n176 = Not(x=w422) -> (.not. x?=w419:bool)
            n177 = Greater?(x=w421, y=w420) -> (0:w423:bool)
            n178 = Select(t=TRUE, s="Считать SIM_SEL", f=w419) -> (s? t:f=w418:bool)
            n179 = And(x=w423, y=w418) -> (x .and. y?=w424:bool)
            n180 = case shown="True" w424 {
              frame False {
              }
              frame True {
                n181 = local read "VCC_counter"() -> (w426:u32)
                n182 = Increment(x=w426) -> (x+1=→"VCC_counter":u32)
              }
            }
          }
        }
      }
      frame #1 {
        w432 = 0
        w441 = 6
        w442 = 6
        w452 = 0
        w453 = 6
        w429 = "\t"
        # "Запись логов"
        n183 = local read "VCC_cur, A"() -> (w450:dbl)
        n184 = local read "DIOD_cur, A"() -> (w443:dbl)
        n185 = local read "DIOD, мA"() -> (w440:dbl)
        n186 = local read "VCC_counter"() -> (w449:u32)
        n187 = local read "VCC_warning"() -> (w444:bool)
        n188 = local read "SEU_Counter"() -> (w434:u32)
        n189 = local read "SEU_warning"() -> (w435:bool)
        n190 = Get Date/Time In Seconds() -> (seconds since 1Jan1904=w456:timestamp)
        n191 = Format Date/Time String(time format string (%c)="%H:%M:%S:%3u", seconds (now)=w456) -> (date/time string=w454:string)  [unwired: 1 in]
        n192 = Number To Fractional String(number=w450, width (-)=w453, precision (6)=w453) -> (F-format string=w448:string)  [unwired: 1 in]
        n193 = Number To Fractional String(number=w443, width (-)=w442, precision (6)=w442) -> (F-format string=w439:string)  [unwired: 1 in]
        n194 = Number To Fractional String(number=w440, width (-)=w441, precision (6)=w441) -> (F-format string=w438:string)  [unwired: 1 in]
        n195 = Number To Fractional String(number=w449, width (-)=w452, precision (6)=w452) -> (F-format string=w437:string)  [unwired: 1 in]
        n196 = Number To Fractional String(number=w434, width (-)=w432, precision (6)=w432) -> (F-format string=w430:string)  [unwired: 1 in]
        n197 = Select(t="!!!", s=w444, f="") -> (s? t:f=w436:string)
        n198 = Select(t="???", s=w435, f="") -> (s? t:f=w427:string)
        n199 = Concatenate Strings(w454, w429, w448, w429, w439, w429, w438, w429, w437, w429, w436, w429, w430, w429, w427, "\r\n") -> (w447:string)
        n200 = Format Into String(initial string=w446, w447) -> (resulting string=w445:refnum<file>)  [unwired: 2 in, 1 out]
      }
      frame #2 {
        n201 = local read "VCC_warning"() -> (w458:bool)
        "SEL" <- w458
        n202 = local read "SEU"() -> (w459:bool)
        n203 = Or(x=w458, y=w459) -> (x .or. y?=w460:bool)
        n204 = case shown="True" w460 {
          tunnel: [w465 w468] -> w463
          tunnel: [w464 w467] -> w462
          tunnel: w461 -> [w464 _]
          frame False {
            n205 = local read "STOP"() -> (w465:bool)
          }
          frame True {
            n206 = flat-sequence {
              tunnel: [FALSE] -> w466
              tunnel: [w474] -> w468
              tunnel: [w473] -> w467
              tunnel: w466 -> [w473]
              frame #0 {
                n207 = local write "POWER"(FALSE ("Power")) -> ()
              }
              frame #1 {
                n208 = Wait (ms)(milliseconds to wait=u32 100 ("Wait_parry, ms")) -> ()  [unwired: 1 out]
              }
              frame #2 {
                n209 = local write "POWER"(TRUE ("Power")) -> ()
              }
              frame #3 {
                n210 = local read "STOP"() -> (w474:bool)
              }
            }
          }
        }
      }
    }
  }
  n211 = flat-sequence {
    tunnel: w17 -> [w479]
    tunnel: w16 -> [_]
    tunnel: w15 -> [_]
    tunnel: w14 -> [_]
    tunnel: w13 -> [w478]
    tunnel: w8 -> [w477]
    tunnel: w1 -> [w475]
    frame #0 {
      # "STOP"
      n212 = Close File(refnum=w475) -> ()  [unwired: 1 in, 2 out]
      n213 = Close File(refnum=w479) -> ()  [unwired: 1 in, 2 out]
      n214 = Wait (ms)(milliseconds to wait=u32 1) -> ()  [unwired: 1 out]
      n215 = call <instrlib>:"niDMM Close.vi"("instrument handle"=w478) -> ()  [unwired: 10 in, 1 out]
      n216 = call <instrlib>:"niScope Close.vi"("instrument handle"=w477) -> ()  [unwired: 14 in, 1 out]
    }
  }
